vi "To Rational.vi"(3 "Number":dbl) -> (0 "Divider":u32, 1 "Numerator":u32)   [LabVIEW 2020, in "LV Tiff.lvlib"]
uses:
  LV Tiff.lvlib
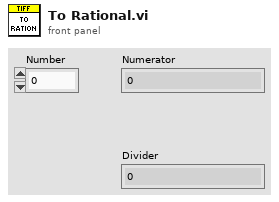
[diagram p1: front panel]
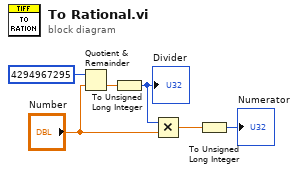
[diagram p0: block diagram]
diagram:
  n1 = Quotient & Remainder(x=u32 4294967295, y="Number") -> (floor(x/y)=w3:dbl)  [unwired: 1 out]
  n2 = To Unsigned Long Integer(number=w3) -> (unsigned 32bit integer=w2:u32)
  "Divider" <- w2
  n3 = Multiply(x=w2, y="Number") -> (x*y=w4:dbl)
  n4 = To Unsigned Long Integer(number=w4) -> (unsigned 32bit integer=→"Numerator":u32)
